vi "Wire Close sessions.vi"(0 "SubVIs Ref":refnum<vi>[](array[refnum]), 11 "error in (no error)":errorcluster) -> (15 "error out":errorcluster)   [LabVIEW 2021, in "Migrator.lvlib"]
uses:
  Migrator.lvlib
  Migrator Reusables/Migrator Reusables.lvlib
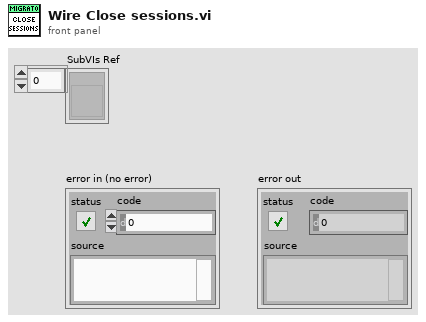
[diagram p1: front panel]
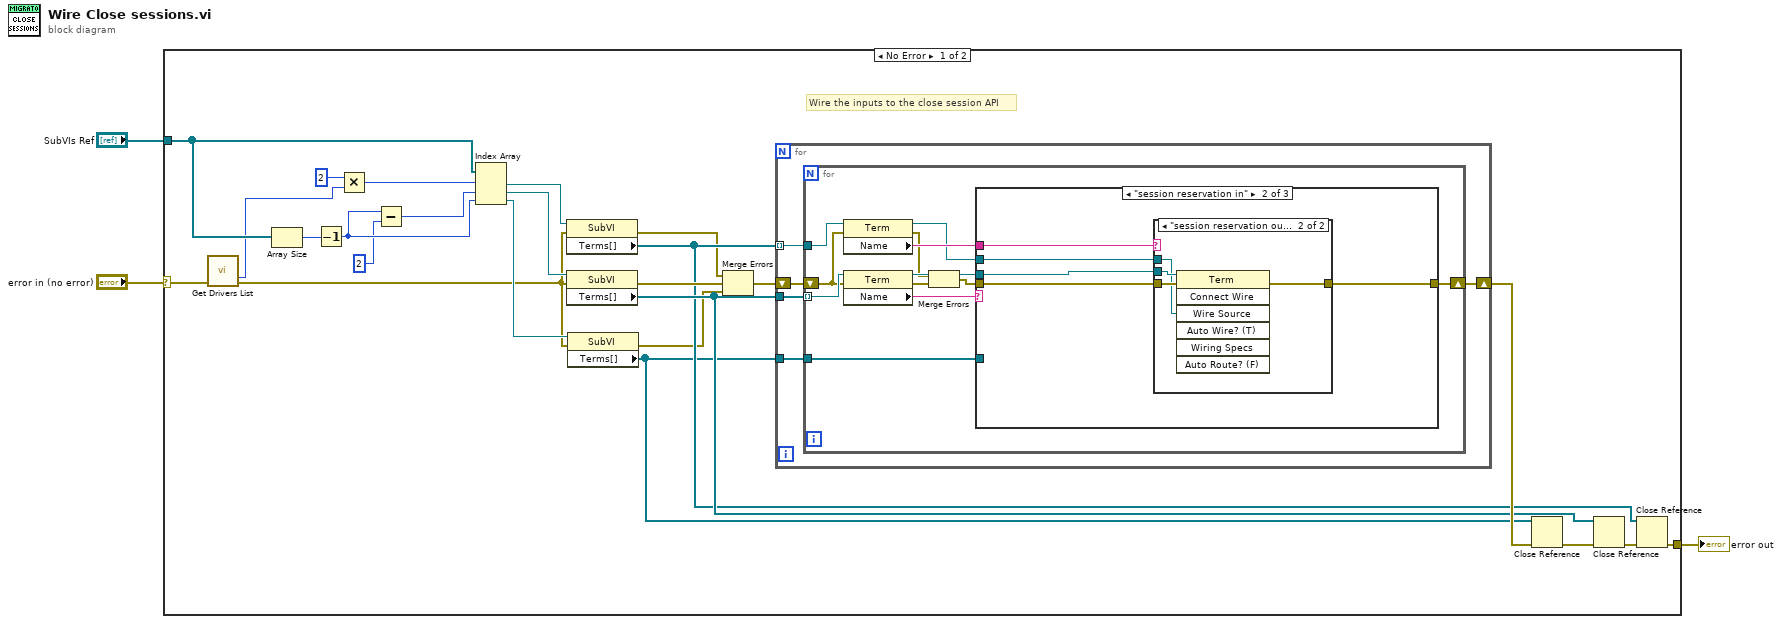
[diagram p0: block diagram]
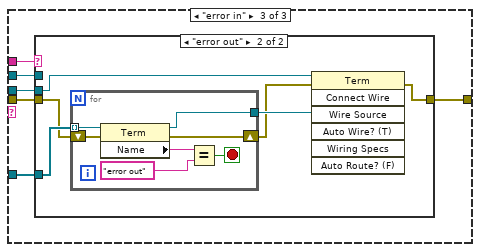
[diagram p4: hidden frame]
diagram:
  n1 = case shown="No Error" "error in (no error)" {
    selector: "error in (no error)" -> [w17 w75]
    tunnel: [w23 w75] -> w3
    tunnel: "SubVIs Ref" -> [w14 _]
    frame No Error {
      # "Wire the inputs to the close session API"
      n2 = call "Get Drivers List.vi"() -> ("Removed Duplicates Size"=w5:i32)  [unwired: 10 in, 5 out]
      n3 = Array Size(array=w14) -> (size(s)=w10:i32)
      n4 = Decrement(x=w10) -> (x-1=w9:i32)
      n5 = Multiply(x=2, y=w5) -> (x*y=w4:i32)
      n6 = Subtract(x=w9, y=2) -> (x-y=w7:i32)
      n7 = Index Array(array=w14, index #1=w4, index #2=w7, index #3=w9) -> (element #1=w20:refnum<vi>, element #2=w19:refnum<vi>, element #3=w18:refnum<vi>)
      n8 = property class="SubVI"(reference=w20, error in=w17) -> (error out=w12:errorcluster, "Terms[]"=w21:refnum<vi>[])  [unwired: 1 out]
      n9 = property class="SubVI"(reference=w19, error in=w17) -> (error out=w26:errorcluster, "Terms[]"=w22:refnum<vi>[])  [unwired: 1 out]
      n10 = property class="SubVI"(reference=w18, error in=w17) -> (error out=w11:errorcluster, "Terms[]"=w16:refnum<vi>[])  [unwired: 1 out]
      n11 = Merge Errors(w12, w26, w11) -> (w13:errorcluster)
      n12 = for {
        tunnel: w21 -> [w30] mode=indexing
        tunnel: w22 -> [w31]
        tunnel: w16 -> [w28]
        shift-right: [w27] -> w25
        shift-left: w13 -> [w29]
        n13 = for {
          tunnel: w31 -> [w42] mode=indexing
          tunnel: w30 -> [w43]
          tunnel: w28 -> [w34]
          shift-right: [w35] -> w27
          shift-left: w29 -> [w41]
          n14 = property class="Term"(reference=w43, error in=w41) -> (reference out=w36:refnum<vi>, error out=w32:errorcluster, "Name"=w40:string)
          n15 = property class="Term"(reference=w42, error in=w41) -> (reference out=w38:refnum<vi>, error out=w37:errorcluster, "Name"=w39:string)
          n16 = Merge Errors(w32, w37) -> (w33:errorcluster)
          n17 = case shown="\"session reservation in\"" w39 {
            tunnel: w40 -> [_ w49 w60]
            tunnel: w38 -> [_ w47 w58]
            tunnel: w33 -> [w44 w48 w59]
            tunnel: [w44 w45 w56] -> w35
            tunnel: w36 -> [_ w46 w57]
            tunnel: w34 -> [_ _ w55]
            frame Default {
            }
            frame "session reservation in" {
              n18 = case shown="\"session reservation out\"" w49 {
                tunnel: w48 -> [w50 w54]
                tunnel: w47 -> [_ w53]
                tunnel: w46 -> [_ w52]
                tunnel: [w50 w51] -> w45
                frame Default {
                }
                frame "session reservation out" {
                  n19 = invoke class="Term" method="Connect Wire"(reference=w53, error in=w54, "Wire Source"=w52) -> (error out=w51:errorcluster)  [unwired: 4 in, 6 out]
                }
              }
            }
            frame "error in" {
              n20 = case shown="\"error out\"" w60 {
                tunnel: w59 -> [w61 w63]
                tunnel: w58 -> [_ w65]
                tunnel: w57 -> [_ _]
                tunnel: [w61 w64] -> w56
                tunnel: w55 -> [_ w67]
                frame Default {
                }
                frame "error out" {
                  n21 = for {
                    tunnel: w67 -> [w74] mode=indexing
                    tunnel: [w69] -> w66
                    shift-right: [w70] -> w62
                    shift-left: w63 -> [w68]
                    stop <- w71 stop-if-true
                    n22 = property class="Term"(reference=w74, error in=w68) -> (reference out=w69:refnum<vi>, error out=w70:errorcluster, "Name"=w73:string)
                    n23 = Equal?(x=w73, y="error out") -> (x = y?=w71:bool)
                  }
                  n24 = invoke class="Term" method="Connect Wire"(reference=w65, error in=w62, "Wire Source"=w66) -> (error out=w64:errorcluster)  [unwired: 4 in, 6 out]
                }
              }
            }
          }
        }
      }
      n25 = Close Reference(reference=w16, error in (no error)=w25) -> (error out=w15:errorcluster)
      n26 = Close Reference(reference=w22, error in (no error)=w15) -> (error out=w24:errorcluster)
      n27 = Close Reference(reference=w21, error in (no error)=w24) -> (error out=w23:errorcluster)
    }
    frame Error {
    }
  }
  "error out" <- w3
